vi "test FIFOs.vi"(8 "error in (no error)":errorcluster, 11 "TestCase in":refnum<class "Configuration Tests.lvclass">=refnum) -> (0 "error out":errorcluster, 3 "TestCase out":refnum<class "Configuration Tests.lvclass">)   [LabVIEW 2021, in "Configuration Tests.lvclass"]
uses:
  Configuration Tests.lvclass
  Classes/Transfer Group/Transfer Group.lvclass
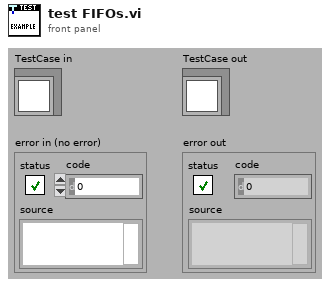
[diagram p1: front panel]
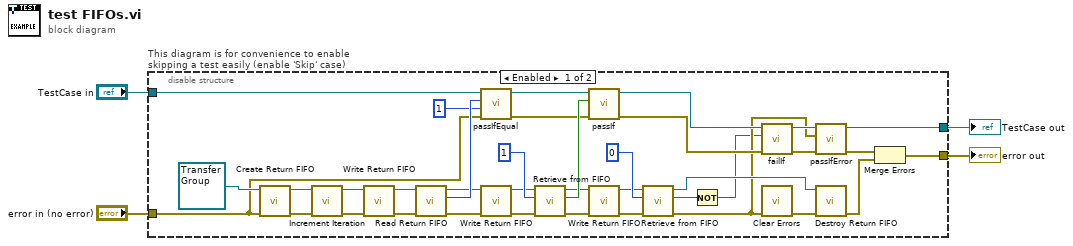
[diagram p0: block diagram]
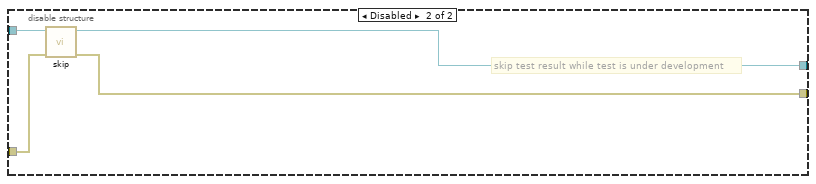
[diagram p2: hidden frame]
diagram:
  n1 = disable-structure "This diagram is for convenience to enable skipping a test easily (enable 'Skip' case)" shown="Enabled" {
    disable-tunnel: "TestCase in" -> [w34 w45]
    disable-tunnel: [w8 w43] -> w1
    disable-tunnel: [w18 w44] -> w3
    disable-tunnel: "error in (no error)" -> [w26 w42]
    frame Enabled {
      n2 = call "Create Return FIFO.vi"("error in (no error)"=w26, "Transfer Group in"=refnum<class "Transfer Group.lvclass"> refnum) -> ("error out"=w41:errorcluster, "Transfer Group out"=w36:refnum<class "Transfer Group.lvclass">)  [unwired: 8 in]
      n3 = call "Increment Iteration.vi"("error in (no error)"=w41, "Transfer Group in"=w36) -> ("error out"=w37:errorcluster, "Transfer Group out"=w35:refnum<class "Transfer Group.lvclass">)  [unwired: 8 in]
      n4 = call "Write Return FIFO.vi"("error in (no error)"=w37, "Transfer Group in"=w35) -> ("error out"=w39:errorcluster, "Transfer Group out"=w40:refnum<class "Transfer Group.lvclass">)  [unwired: 7 in, 1 out]
      n5 = call "Read Return FIFO.vi"("error in (no error)"=w39, "Transfer Group in"=w40) -> ("error out"=w27:errorcluster, "Transfer Group iteration"=w32:u64, "Transfer Group out"=w16:refnum<class "Transfer Group.lvclass">)  [unwired: 6 in, 1 out]
      n6 = call-dynamic "passIfEqual.vi"("error in (no error)"=w26, "y"=u64 1 ("Transfer Group iteration"), "x"=w32, "TestCase in"=w34) -> ("error out"=w19:errorcluster, "TestCase out"=w33:refnum<class "Configuration Tests.lvclass">)  [unwired: 6 in]
      n7 = call "Write Return FIFO.vi"("error in (no error)"=w27, "Transfer Group in"=w16) -> ("error out"=w17:errorcluster, "Transfer Group out"=w15:refnum<class "Transfer Group.lvclass">)  [unwired: 7 in, 1 out]
      n8 = call "Retrieve from FIFO.vi"("error in (no error)"=w17, "expected iteration"=u64 1, "Transfer Group in"=w15) -> ("error out"=w30:errorcluster, "ready"=w24:bool, "Transfer Group out"=w13:refnum<class "Transfer Group.lvclass">)  [unwired: 5 in, 1 out]
      n9 = call-dynamic "passIf.vi"("error in (no error)"=w19, "pass"=w24, "TestCase in"=w33) -> ("error out"=w20:errorcluster, "TestCase out"=w25:refnum<class "Configuration Tests.lvclass">)  [unwired: 7 in]
      n10 = call "Write Return FIFO.vi"("error in (no error)"=w30, "Transfer Group in"=w13) -> ("error out"=w14:errorcluster, "Transfer Group out"=w12:refnum<class "Transfer Group.lvclass">)  [unwired: 7 in, 1 out]
      n11 = call "Retrieve from FIFO.vi"("error in (no error)"=w14, "expected iteration"=u64 0, "Transfer Group in"=w12) -> ("error out"=w6:errorcluster, "ready"=w22:bool, "Transfer Group out"=w23:refnum<class "Transfer Group.lvclass">)  [unwired: 5 in, 1 out]
      n12 = Not(x=w22) -> (.not. x?=w5:bool)
      n13 = call-dynamic "failIf.vi"("error in (no error)"=w20, "fail"=w5, "TestCase in"=w25) -> ("error out"=w7:errorcluster, "TestCase out"=w9:refnum<class "Configuration Tests.lvclass">)  [unwired: 7 in]
      n14 = call <vilib>:"Clear Errors.vi"("error in (no error)"=w6) -> ("error out"=w11:errorcluster)  [unwired: 5 in, 1 out]
      n15 = call-dynamic "passIfError.vi"("error in (no error)"=w7, "error"=w6, "TestCase in"=w9) -> ("error out"=w10:errorcluster, "TestCase out"=w8:refnum<class "Configuration Tests.lvclass">)  [unwired: 7 in]
      n16 = call "Destroy Return FIFO.vi"("error in (no error)"=w11, "Transfer Group in"=w23) -> ("error out"=w28:errorcluster)  [unwired: 8 in, 1 out]
      n17 = Merge Errors(w10, w28) -> (w18:errorcluster)
    }
    frame Disabled {
      # "skip test result while test is under development"
      n18 = call <vilib>:"skip.vi"("error in (no error)"=w42, "TestCase in"=w45) -> ("error out"=w44:errorcluster, "TestCase out"=w43:refnum<class "Configuration Tests.lvclass">)  [unwired: 8 in]
    }
  }
  "error out" <- w3
  "TestCase out" <- w1
